vi "_getConnectionFromGUID.vi"(8 "error in (no error)":errorcluster, 10 "GUID":string, 11 "tWorkerController in":refnum<class "tWorkerController.lvclass">) -> (0 "error out":errorcluster, 2 "TCP Connection":T1, 3 "tWorkerController out":refnum<class "tWorkerController.lvclass">)   [LabVIEW 2013, in "tWorkerController.lvlib" / "tWorkerController.lvclass"]
uses:
  tWorkerController.lvclass
  _tcpConnection.ctl
  <vilib>/ActorFramework/Message Enqueuer/Message Enqueuer.lvclass
  tWorkerController.lvclass/tWorkerController.ctl
  _status.ctl
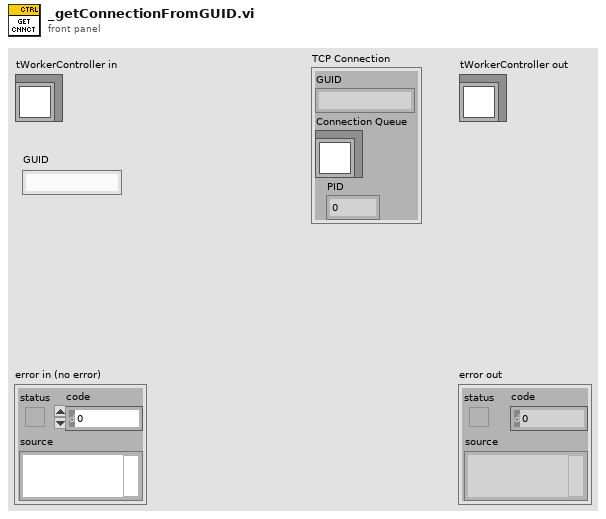
[diagram p1: front panel]
types:
  T1 = typedef "tWorkerController.lvlib/tWorkerController.lvclass/_tcpConnection.ctl" = cluster{"GUID":string, "Connection Queue":refnum<class "Message Enqueuer.lvclass">, "PID":i64}
  T2 = typedef "tWorkerController.lvlib/tWorkerController.lvclass/_status.ctl" = enum16{"Problem Launching Worker", "Worker Not Found", "Test Not In Library", "Connection Not Found"}
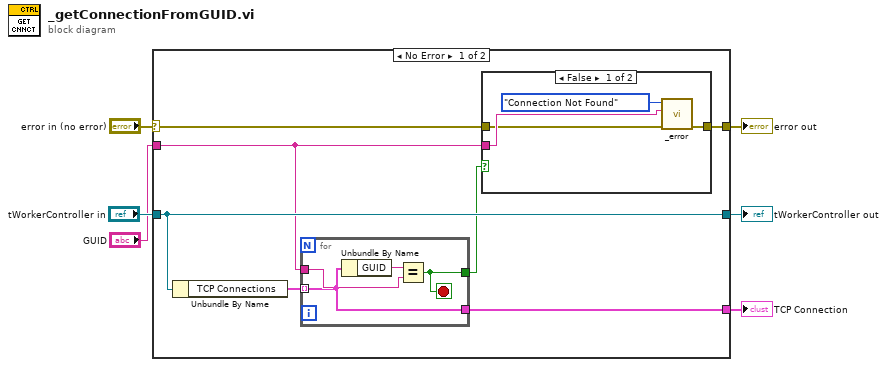
[diagram p0: block diagram]
diagram:
  n1 = case shown="No Error" "error in (no error)" {
    selector: "error in (no error)" -> [w8 w24]
    tunnel: [w10 w24] -> w5
    tunnel: [w13 w23] -> w3
    tunnel: "tWorkerController in" -> [w13 w23]
    tunnel: "GUID" -> [w9 _]
    tunnel: [w7 _] -> w1
    frame No Error {
      n2 = Unbundle By Name(w13) -> ("TCP Connections"=w12:T1[])
      n3 = for {
        tunnel: w12 -> [w19] mode=indexing
        tunnel: w9 -> [w21]
        tunnel: [w20] -> w11
        tunnel: [w19] -> w7
        stop <- w20 stop-if-true
        n4 = Unbundle By Name(w19) -> ("GUID"=w22:string)
        n5 = Equal?(x=w22, y=w21) -> (x = y?=w20:bool)
      }
      n6 = case shown="False" w11 {
        tunnel: [w17 w18] -> w10
        tunnel: w9 -> [w16 _]
        tunnel: w8 -> [w14 w18]
        frame False {
          n7 = call "_error.vi"("error in (no error)"=w14, "Additional message"=w16, "Status"=_status."Connection Not Found") -> ("error out"=w17:errorcluster)  [unwired: 8 in]
        }
        frame True {
        }
      }
    }
    frame Error {
    }
  }
  "error out" <- w5
  "tWorkerController out" <- w3
  "TCP Connection" <- w1
